vi "MC5e Save_Config_XML.vi"(8 "error In":errorcluster, 9 "Control References[]":refnum<vi>[](array[refnum]), 10 "Cancelled?":bool, 11 "selected path":path) -> (0 "error out":errorcluster)   [LabVIEW 2020]
uses:
  MC5e Control_Info_Cluster.ctl
  NI-source-code/NI Custom VIs/Utilities/Security/Cryptographic Services/SHA256/SHA256.lvlib
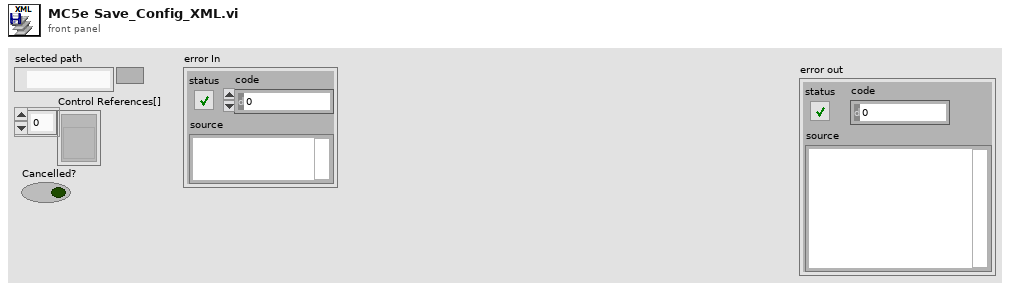
[diagram p1: front panel]
types:
  T1 = cluster{"SHA256 Hash of Controls":string, "Controls Array XML":string}
  T2 = typedef "MC5e Control_Info_Cluster.ctl" = cluster{"reference":refnum<vi>, "Class Name":string, "Label.Text":string, "Value":variant, "Control Index":i32}
  T3 = enum16{"open", "replace", "create", "open or create", "replace or create", "replace or create with confirmation"}
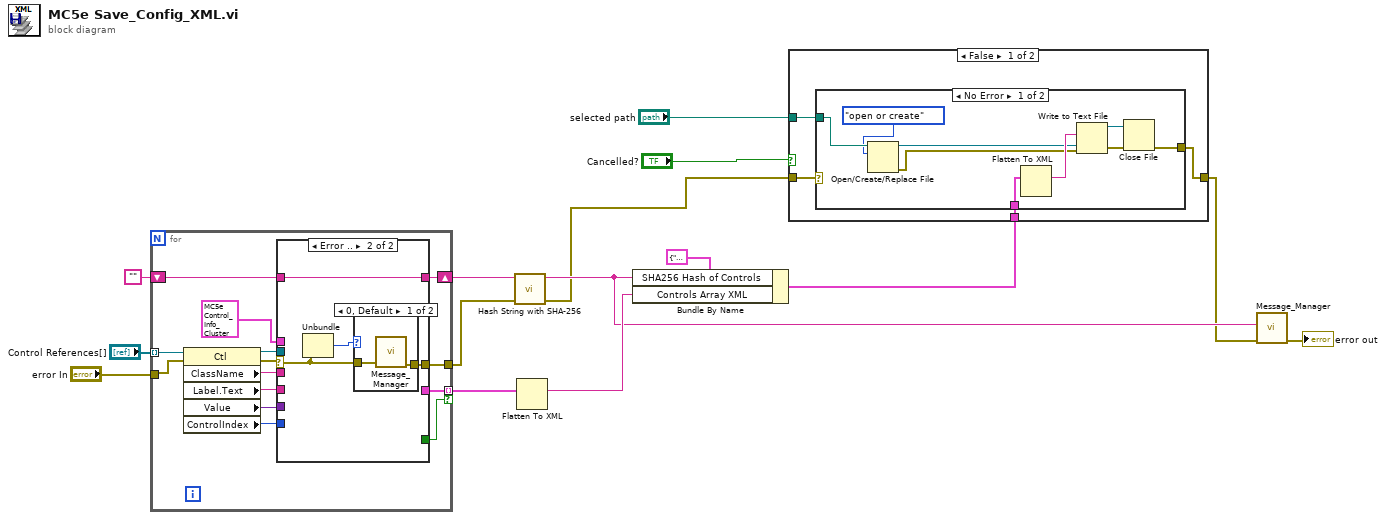
[diagram p0: block diagram]
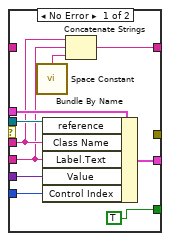
[diagram p2: hidden frame]
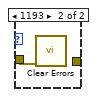
[diagram p3: hidden frame]
diagram:
  n1 = for {
    tunnel: [w24] -> w6 mode=indexing if=w20
    shift-right: [w21] -> w7
    shift-left: "" -> [w19]
    tunnel: "Control References[]" -> [w18] mode=indexing
    tunnel: "error In" -> [w17]
    tunnel: [w16] -> w4
    n2 = property class="Ctl"(reference=w18, error in=w17) -> (reference out=w29:refnum<vi>, error out=w23:errorcluster, "ClassName"=w28:string, "Label.Text"=w27:string, "Value"=w26:variant, "ControlIndex"=w25:i32)
    n3 = case shown="Error .." w23 {
      selector: w23 -> [_ w42]
      tunnel: w29 -> [w39 _]
      tunnel: w28 -> [w33 _]
      tunnel: w27 -> [w32 _]
      tunnel: w26 -> [w38 _]
      tunnel: w25 -> [w37 _]
      tunnel: [w36 _] -> w24
      tunnel: [TRUE _] -> w20
      tunnel: T2 {"reference"=refnum, "Class Name"="", "Label.Text"="", "Value"=variant, "Control Index"=0} -> [w34 _]
      tunnel: [w31 w43] -> w21
      tunnel: w19 -> [_ w43]
      tunnel: [_ w40] -> w16
      frame No Error {
        n4 = call <vilib>:"Space Constant.vi"() -> ("String"=w30:string)
        n5 = Bundle By Name(cluster=w34, "reference"=w39, "Class Name"=w33, "Label.Text"=w32, "Value"=w38, "Control Index"=w37) -> (w36:T2)
        n6 = Concatenate Strings(w33, w32, w30) -> (w31:string)
      }
      frame Error {
        n7 = Unbundle(w42) -> ("code"=w41:i32)  [unwired: 2 out]
        n8 = case shown="0, Default" w41 {
          tunnel: w42 -> [w45 w46]
          tunnel: [w44 _] -> w40
          frame 0, Default {
            n9 = call "Message_Manager.vi"("error in"=w45) -> ("error out"=w44:errorcluster)  [unwired: 6 in, 4 out]
          }
          frame 1193 {
            n10 = call <vilib>:"Clear Errors.vi"("error in (no error)"=w46) -> ()  [unwired: 5 in, 2 out]
          }
        }
      }
    }
  }
  n11 = call "Hash String with SHA-256.vi"("error In"=w4, "String to Encode"=w7) -> ("error Out"=w3:errorcluster, "Hash String"=w10:string)  [unwired: 8 in]
  n12 = Flatten To XML(6:w6) -> (2:w13:string)
  n13 = Bundle By Name(cluster=T1 {"SHA256 Hash of Controls"="", "Controls Array XML"=""}, "SHA256 Hash of Controls"=w10, "Controls Array XML"=w13) -> (w12:T1)
  n14 = case shown="False" "Cancelled?" {
    tunnel: [w50 w61] -> w9
    tunnel: w12 -> [w49 _]
    tunnel: w3 -> [w47 w61]
    tunnel: "selected path" -> [w48 _]
    frame False {
      n15 = case shown="No Error" w47 {
        selector: w47 -> [_ w60]
        tunnel: [w59 w60] -> w50
        tunnel: w49 -> [w57 _]
        tunnel: w48 -> [w54 _]
        frame No Error {
          n16 = Open/Create/Replace File(file path (use dialog)=w54, operation (0:open)=T3."open or create") -> (refnum out=w53:refnum<file>, error out=w51:errorcluster)  [unwired: 4 in, 1 out]
          n17 = Flatten To XML(6:w57) -> (2:w56:string)
          n18 = Write to Text File(file (use dialog)=w53, text=w56, error in=w51) -> (refnum out=w58:refnum<file>, error out=w55:errorcluster)  [unwired: 1 in, 1 out]
          n19 = Close File(refnum=w58, error in=w55) -> (error out=w59:errorcluster)  [unwired: 1 out]
        }
        frame Error {
        }
      }
    }
    frame True {
    }
  }
  n20 = call "Message_Manager.vi"("error in"=w9, "New Entry"=w10) -> ("error out"=→"error out":errorcluster)  [unwired: 5 in, 4 out]
